vi "Check Expected Heartbeat.vi"(8 "error in":errorcluster, 11 "CANopen Master in":refnum<class "CANopen Master.lvclass">) -> (0 "error out":errorcluster, 1 "Emergency?":bool[](array[boolean]), 2 "Nodes":u8[](array[numeric]), 3 "CANopen Master out":refnum<class "CANopen Master.lvclass">)   [LabVIEW 2024]
uses:
  CANopen Master.lvclass/CANopen Master.ctl
  CANopen Master.lvclass
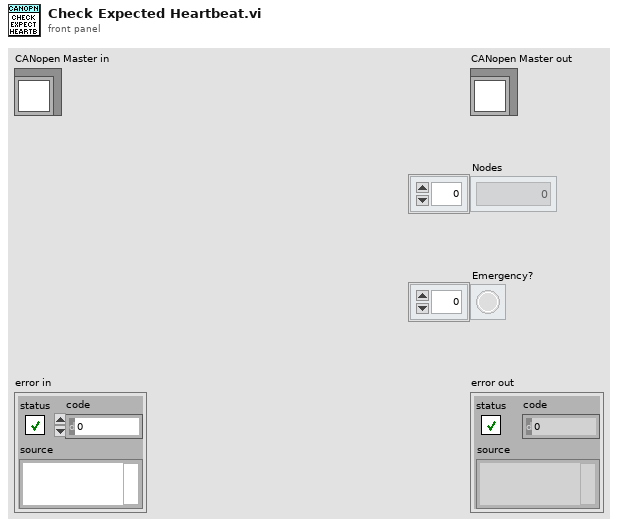
[diagram p1: front panel]
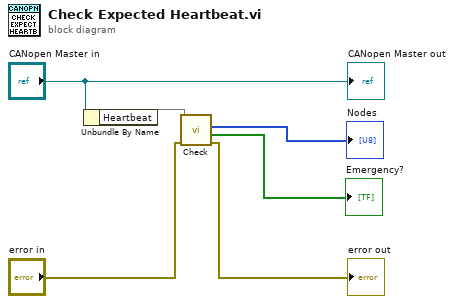
[diagram p0: block diagram]
diagram:
  n1 = Unbundle By Name("CANopen Master in") -> ("Heartbeat"=w5)
  n2 = call "Check.vi"("Error In"="error in", "reference in"=w5) -> ("Error Out"=→"error out":errorcluster, "Emergency?"=→"Emergency?":bool[], "Nodes"=→"Nodes":u8[])  [unwired: 6 in, 1 out]
  "CANopen Master out" <- "CANopen Master in"
